vi "Get Row of reflection.vi"(8 "error in (no error)":errorcluster, 10 "Start point":u64, 11 "Proto in":refnum<class "Group.lvclass">) -> (0 "error out":errorcluster, 2 "Numeric":u64, 3 "Proto out":refnum<class "Group.lvclass">)   [LabVIEW 2020, in "Group.lvclass"]
uses:
  Group.lvclass
  Group.lvclass/Group.ctl
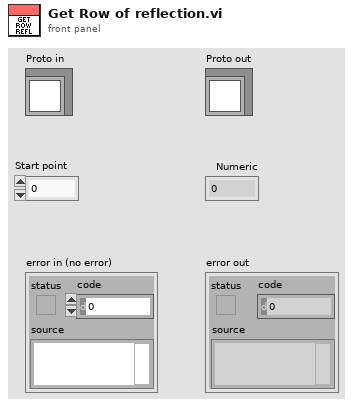
[diagram p1: front panel]
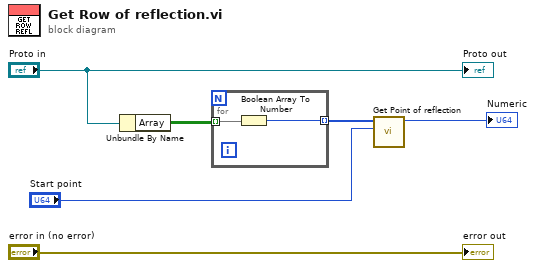
[diagram p0: block diagram]
diagram:
  n1 = Unbundle By Name("Proto in") -> ("Array"=w4:bool[][])
  n2 = for {
    tunnel: w4 -> [w8] mode=indexing
    tunnel: [w7] -> w3 mode=indexing
    n3 = Boolean Array To Number(Boolean array=w8) -> (number=w7:u32)
  }
  n4 = call "Get Point of reflection.vi"("Start point"="Start point", "Array in"=w3) -> ("Numeric"=→"Numeric":u64)  [unwired: 9 in]
  "error out" <- "error in (no error)"
  "Proto out" <- "Proto in"
